vi "dt_powers.vi"(11 "feedback_time (ms)":fxp<+,16,1>) -> (0 "dt^3/2":fxp<+,48,1>, 1 "dt^3":fxp<+,48,1>, 2 "dt^4/4":fxp<+,64,4>, 3 "dt^2":fxp<+,32,2> format="%#_13g", 4 "output valid":bool)   [LabVIEW 2020]
uses:
  <vilib>/rvi/FXPMathLib/FxpMul/XNode/nifxpmath_Multiplier.xnode
  <vilib>/rvi/FXPMathLib/sim/FxpSim.dll
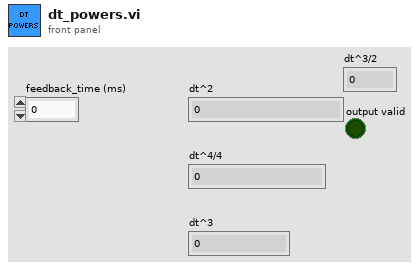
[diagram p1: front panel]
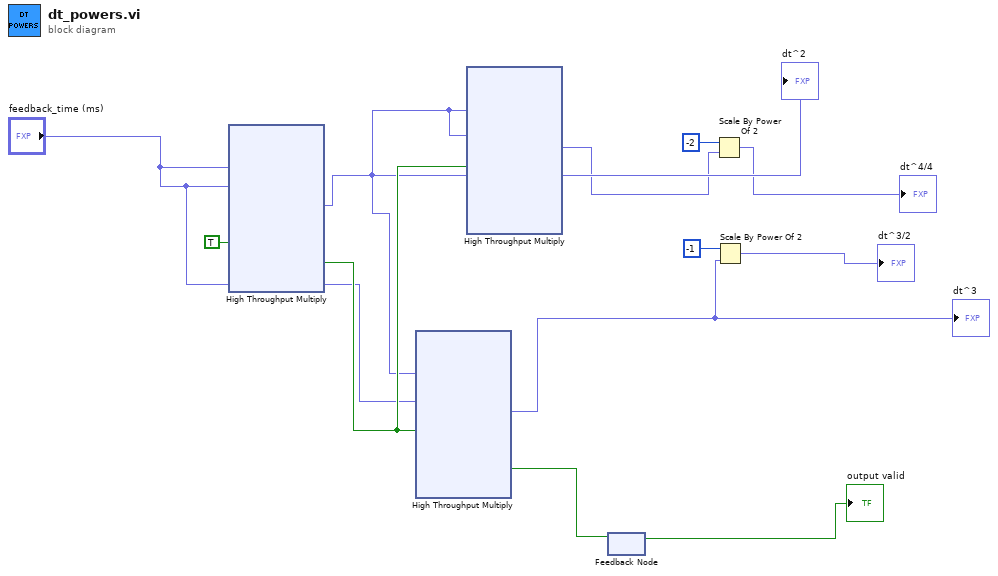
[diagram p0: block diagram]
diagram:
  n1 = xnode "High Throughput Multiply"("x"="feedback_time (ms)", "y"="feedback_time (ms)", "input valid"=TRUE) -> ("x*y"=w9:fxp<+,32,2>, "output valid"=w12:bool)  [unwired: 1 in, 1 out]
  "dt^2" <- w9
  n2 = xnode "High Throughput Multiply"("x"=w9, "y"="feedback_time (ms)", "input valid"=w12) -> ("x*y"=w5:fxp<+,48,1>, "output valid"=w3:bool)  [unwired: 1 in, 1 out]
  "dt^3" <- w5
  n3 = xnode "High Throughput Multiply"("x"=w9, "y"=w9, "input valid"=w12) -> ("x*y"=w8:fxp<+,64,4>)  [unwired: 1 in, 2 out]
  n4 = feedback-in #1(w3) -> ()
  n5 = feedback #1() -> (→"output valid":bool)  [unwired: 1 in]
  n6 = Scale By Power Of 2(n=i16 -2, x=w8) -> (x*2^n=→"dt^4/4":fxp<+,64,4>)
  n7 = Scale By Power Of 2(n=i16 -1, x=w5) -> (x*2^n=→"dt^3/2":fxp<+,48,1>)
